vi "IPC-Core-ModbusModule20150814.vi"(8 "error in":errorcluster, 9 "ErrorQRef":refnum<queue>, 10 "ModbusQRef":refnum<queue>, 11 "CmdQRef":refnum<queue>) -> (0 "error out":errorcluster)   [LabVIEW 2014]
uses:
  Configuration-Global.vi
panel:
  in  "Modbus Module State":enum16{"Start", "Pause", "Exit"}(ring)
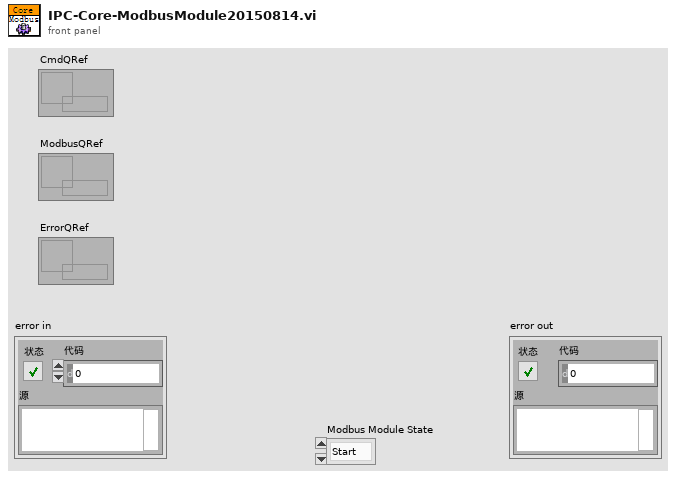
[diagram p1: front panel]
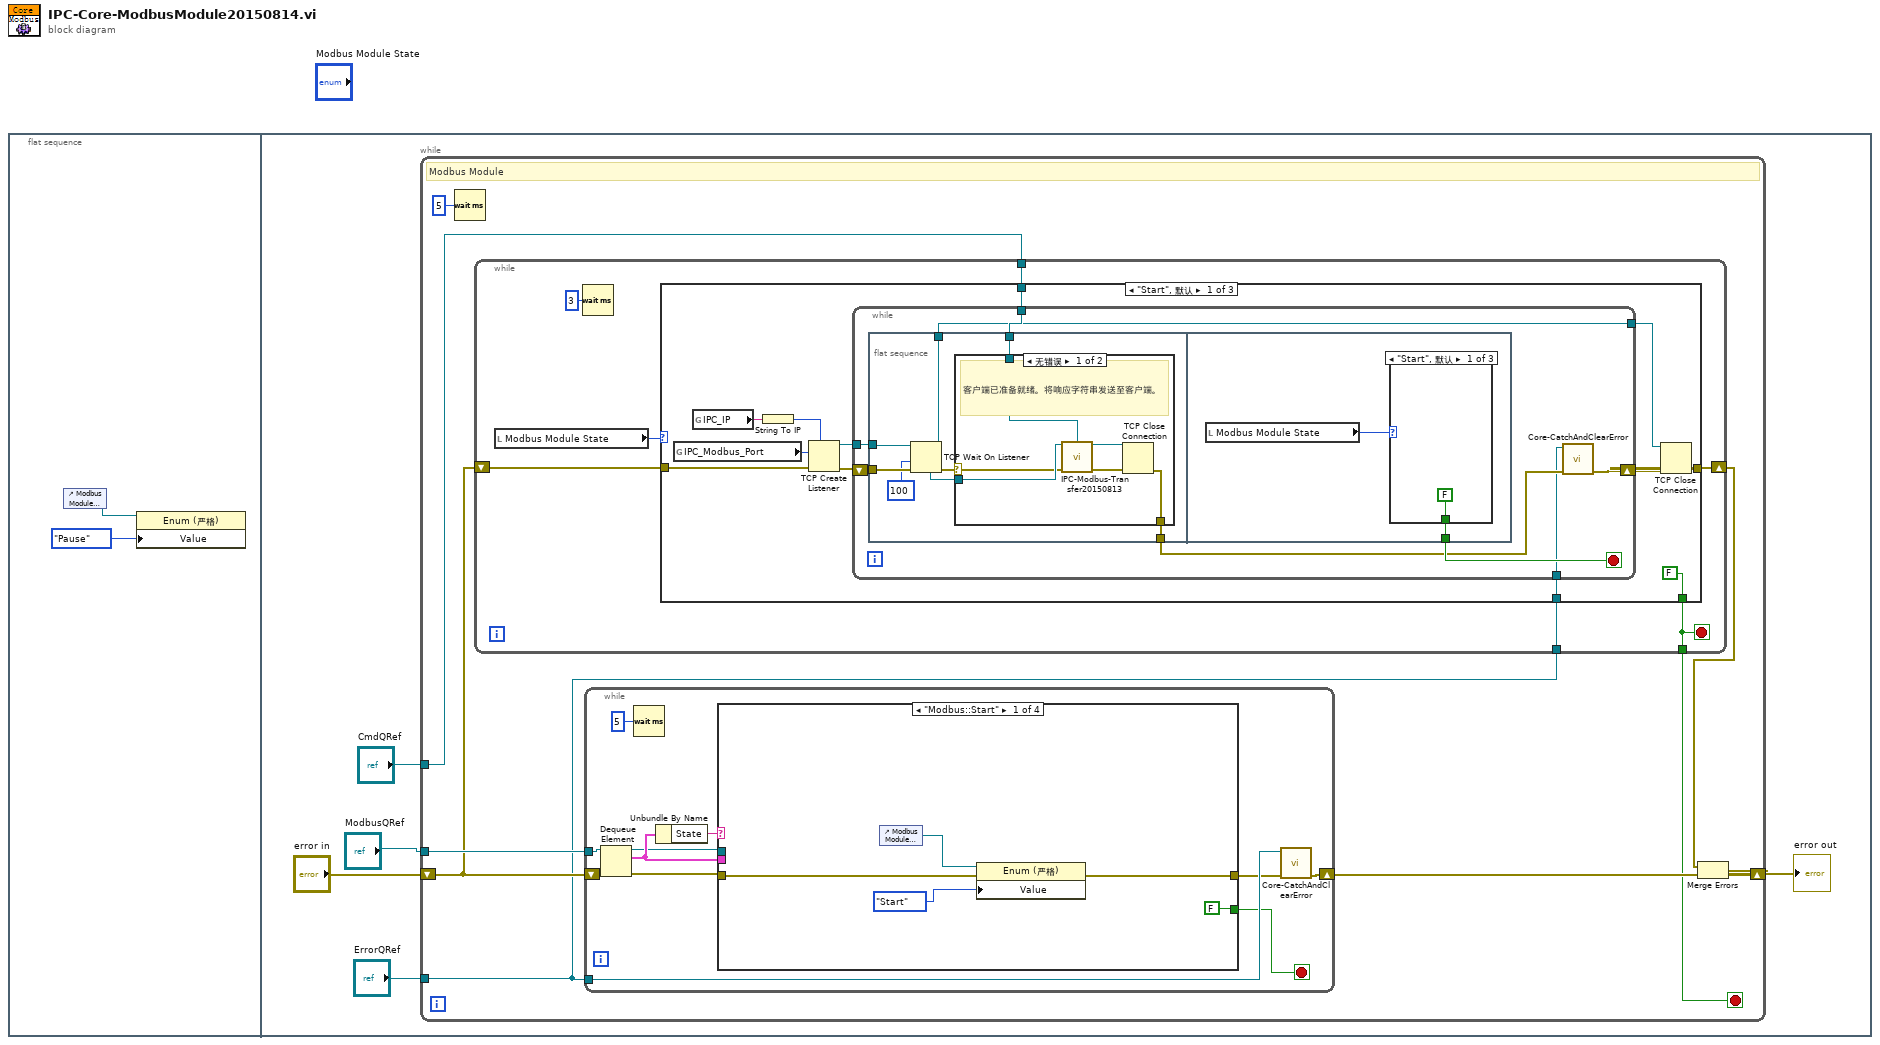
[diagram p0: block diagram]
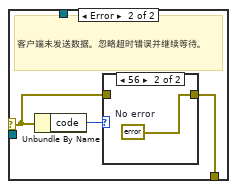
[diagram p2: hidden frame]
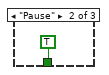
[diagram p4: hidden frame]
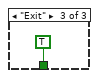
[diagram p5: hidden frame]
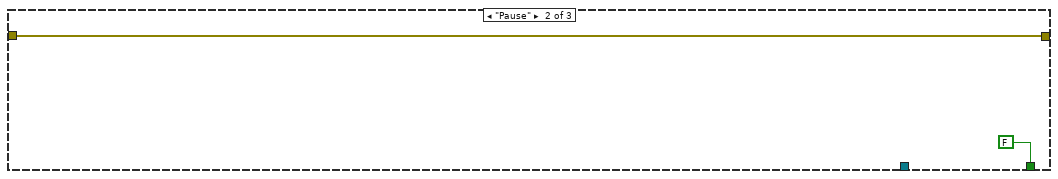
[diagram p6: hidden frame]
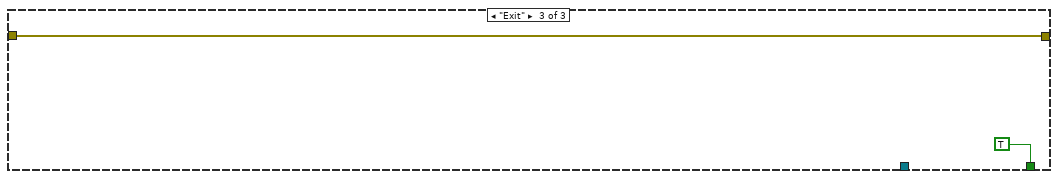
[diagram p7: hidden frame]
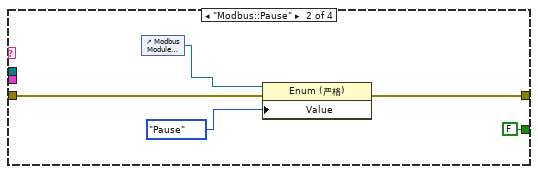
[diagram p8: hidden frame]
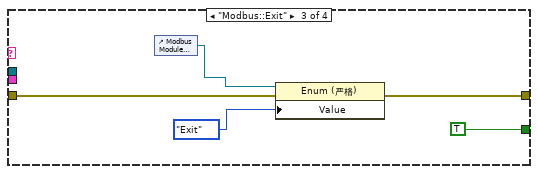
[diagram p9: hidden frame]
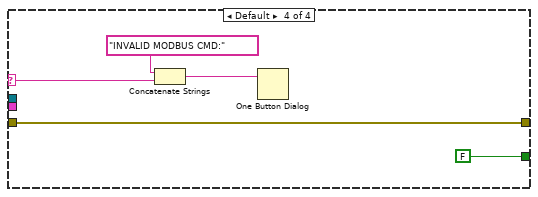
[diagram p10: hidden frame]
diagram:
  n1 = flat-sequence {
    frame #0 {
      n2 = control-ref of="Modbus Module State"() -> (w1:refnum<vi>)
      n3 = property class="Enum (严格)"(reference=w1, "Value"=enum16{"Start", "Pause", "Exit"}."Pause" ("枚举")) -> ()  [unwired: 1 in, 2 out]
    }
    frame #1 {
      n4 = while {
        shift-right: [w12] -> w4
        shift-left: "error in" -> [w11]
        tunnel: "ErrorQRef" -> [w10]
        tunnel: "ModbusQRef" -> [w15]
        tunnel: "CmdQRef" -> [w14]
        stop <- w8 stop-if-true
        # "Modbus Module"
        n5 = Wait (ms)(milliseconds to wait=u32 5 ("等待时间（毫秒）")) -> ()  [unwired: 1 out]
        n6 = while {
          tunnel: w14 -> [w23]
          shift-right: [w22] -> w9
          shift-left: w11 -> [w19]
          tunnel: w10 -> [w18]
          tunnel: [w17] -> w8
          stop <- w17 stop-if-true
          n7 = local read "Modbus Module State"() -> (w20:enum16{"Start", "Pause", "Exit"})
          n8 = Wait (ms)(milliseconds to wait=u32 3 ("等待时间（毫秒）")) -> ()  [unwired: 1 out]
          n9 = case shown="\"Start\", 默认" w20 {
            tunnel: w23 -> [w35 _ _]
            tunnel: [w34 w69 w70] -> w22
            tunnel: w19 -> [w26 w69 w70]
            tunnel: [FALSE FALSE TRUE] -> w17
            tunnel: w18 -> [w24 _ _]
            frame "Start", Default {
              n10 = global read "Configuration-Global.vi" "IPC_Modbus_Port"() -> (w29:i32)
              n11 = global read "Configuration-Global.vi" "IPC_IP"() -> (w27:string)
              n12 = String To IP(1:w27) -> (0:w28:u32)
              n13 = TCP Create Listener(7:w28, 8:w26, 10:w29) -> (0:w30:errorcluster, 3:w31:refnum<k5>)  [unwired: 2 in, 1 out]
              n14 = while {
                tunnel: w35 -> [w42]
                tunnel: w31 -> [w41]
                tunnel: [w39] -> w33
                shift-right: [w37] -> w32
                shift-left: w30 -> [w40]
                tunnel: w24 -> [w36]
                stop <- w43 stop-if-true
                n15 = flat-sequence {
                  tunnel: w42 -> [w51]
                  tunnel: w41 -> [w50]
                  tunnel: w40 -> [w49]
                  tunnel: [w48] -> w39
                  tunnel: [w46] -> w38
                  tunnel: [w64] -> w43
                  frame #0 {
                    n16 = TCP Wait On Listener(8:w49, 9:100 ("超时毫秒（一直等待:-1）"), 11:w50) -> (0:w45:errorcluster, 3:w48:refnum<k5>, 4:w47:refnum<k5>)  [unwired: 1 in, 2 out]
                    n17 = case shown="无错误" w45 {
                      selector: w45 -> [w52 w59]
                      tunnel: w51 -> [w57 _]
                      tunnel: w47 -> [w56 _]
                      tunnel: [w53 w58] -> w46
                      frame No Error {
                        # "客户端已准备就绪。将响应字符串发送至客户端。"
                        n18 = call "IPC-Modbus-Transfer20150813.vi"("connection ID in"=w56, "CmdQRef"=w57, "错误输入（无错误）"=w52) -> ("connection ID out"=w55:refnum<k5>, "错误输出"=w54:errorcluster)  [unwired: 11 in]
                        n19 = TCP Close Connection(connection ID=w55, error in (no error)=w54) -> (error out=w53:errorcluster)  [unwired: 1 in, 1 out]
                      }
                      frame Error {
                        # "客户端未发送数据。忽略超时错误并继续等待。"
                        n20 = Unbundle By Name(w59) -> ("code"=w60:i32)
                        n21 = case shown="56" w60 {
                          tunnel: w59 -> [w61 _]
                          tunnel: [w61 w62] -> w58
                          frame Default {
                          }
                          frame 56 {
                            w62 = errorcluster {"status"=FALSE, "code"=0, "source"=""}  # No error
                          }
                        }
                      }
                    }
                  }
                  frame #1 {
                    n22 = local read "Modbus Module State"() -> (w63:enum16{"Start", "Pause", "Exit"})
                    n23 = case shown="\"Start\", 默认" w63 {
                      tunnel: [FALSE TRUE TRUE] -> w64
                      frame "Start", Default {
                      }
                      frame "Pause" {
                      }
                      frame "Exit" {
                      }
                    }
                  }
                }
                n24 = call "Core-CatchAndClearError.vi"("error in (no error)"=w38, "ErrorQ"=w36) -> ("error out"=w37:errorcluster)  [unwired: 7 in]
              }
              n25 = TCP Close Connection(connection ID=w33, error in (no error)=w32) -> (error out=w34:errorcluster)  [unwired: 1 in, 1 out]
            }
            frame "Pause" {
            }
            frame "Exit" {
            }
          }
        }
        n26 = while {
          tunnel: w10 -> [w78]
          tunnel: w15 -> [w75]
          shift-right: [w79] -> w13
          shift-left: w11 -> [w82]
          stop <- w73 stop-if-true
          n27 = Dequeue Element(queue=w75, error in (no error)=w82) -> (queue out=w74:refnum<queue>, element=w76:cluster{"Data":variant, "State":string}, error out=w81:errorcluster)  [unwired: 1 in, 1 out]
          n28 = Wait (ms)(milliseconds to wait=u32 5 ("等待时间（毫秒）")) -> ()  [unwired: 1 out]
          n29 = Unbundle By Name(w76) -> ("State"=w80:string)
          n30 = case shown="\"Modbus::Start\"" w80 {
            selector: w80 -> [_ _ _ w99]
            tunnel: w81 -> [w86 w91 w94 w102]
            tunnel: [w85 w90 w93 w102] -> w77
            tunnel: w76 -> [_ _ _ _]
            tunnel: w74 -> [_ _ _ _]
            tunnel: [FALSE FALSE TRUE FALSE] -> w73
            frame "Modbus::Start" {
              n31 = control-ref of="Modbus Module State"() -> (w84:refnum<vi>)
              n32 = property class="Enum (严格)"(reference=w84, error in=w86, "Value"=enum16{"Start", "Pause", "Exit"}."Start" ("枚举")) -> (error out=w85:errorcluster)  [unwired: 1 out]
            }
            frame "Modbus::Pause" {
              n33 = control-ref of="Modbus Module State"() -> (w89:refnum<vi>)
              n34 = property class="Enum (严格)"(reference=w89, error in=w91, "Value"=enum16{"Start", "Pause", "Exit"}."Pause" ("枚举")) -> (error out=w90:errorcluster)  [unwired: 1 out]
            }
            frame "Modbus::Exit" {
              n35 = control-ref of="Modbus Module State"() -> (w96:refnum<vi>)
              n36 = property class="Enum (严格)"(reference=w96, error in=w94, "Value"=enum16{"Start", "Pause", "Exit"}."Exit" ("枚举")) -> (error out=w93:errorcluster)  [unwired: 1 out]
            }
            frame Default {
              n37 = Concatenate Strings("INVALID MODBUS CMD:", w99) -> (w100:string)
              n38 = One Button Dialog(message=w100) -> ()  [unwired: 1 in, 1 out]
            }
          }
          n39 = call "Core-CatchAndClearError.vi"("error in (no error)"=w77, "ErrorQ"=w78) -> ("error out"=w79:errorcluster)  [unwired: 7 in]
        }
        n40 = Merge Errors(w9, w13) -> (w12:errorcluster)
      }
      "error out" <- w4
    }
  }
